vi "RS_SMBV100A_Message.vi"(3 "Boolean":bool, 4 "error in":errorcluster, 5 "F button name (\"Cancel\")":string, 6 "T button name (\"OK\")":string, 7 "message":string) -> (0 "error IO":errorcluster, 2 "MODE":string)   [LabVIEW 2018]
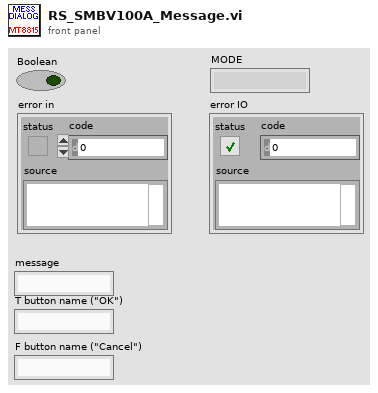
[diagram p1: front panel]
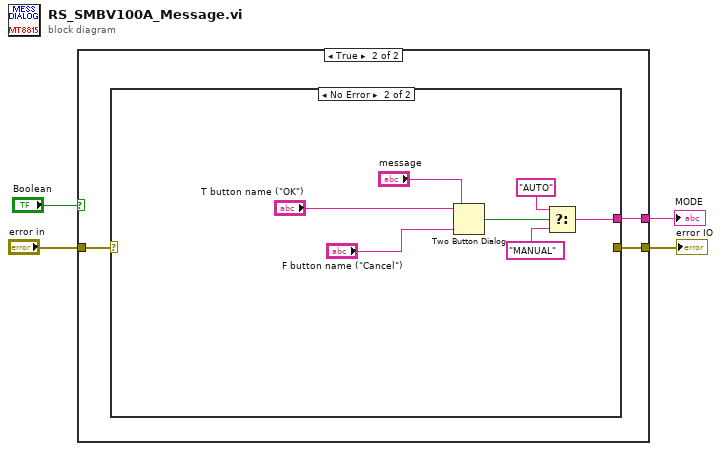
[diagram p0: block diagram]
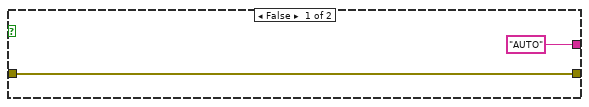
[diagram p2: hidden frame]
diagram:
  n1 = case shown="True" "Boolean" {
    tunnel: "error in" -> [w5 w9]
    tunnel: [w5 w8] -> w3
    tunnel: ["AUTO" w7] -> w2
    frame False {
    }
    frame True {
      n2 = case shown="No Error" w9 {
        selector: w9 -> [w10 _]
        tunnel: [w10 _] -> w8
        tunnel: [_ w14] -> w7
        frame Error {
        }
        frame No Error {
          n3 = Two Button Dialog(message="message", 1:"F button name (\"Cancel\")", 2:"T button name (\"OK\")") -> (T button?=w17:bool)
          n4 = Select(t="AUTO", s=w17, f="MANUAL") -> (s? t:f=w14:string)
        }
      }
    }
  }
  "error IO" <- w3
  "MODE" <- w2
